vi "Create NIVS Custom Device API.vi"(8 "error in":errorcluster, 9 "Custom Device Item Ref":u64 format="%.0x") -> (0 "error out":errorcluster, 3 "NIVS Custom Device API out":refnum<class "NIVS Custom Device API.lvclass">)   [LabVIEW 2026, in "Template Engine.lvlib" / "NIVS Custom Device API.lvclass"]
uses:
  NIVS Custom Device API.lvclass
  NIVS Custom Device API.lvclass/NIVS Custom Device API.ctl
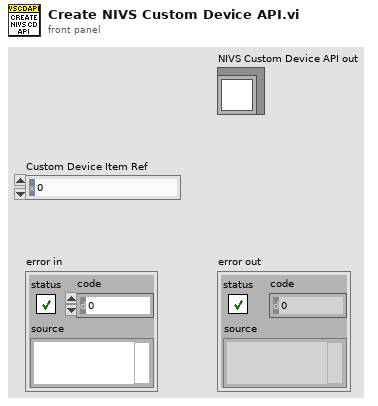
[diagram p1: front panel]
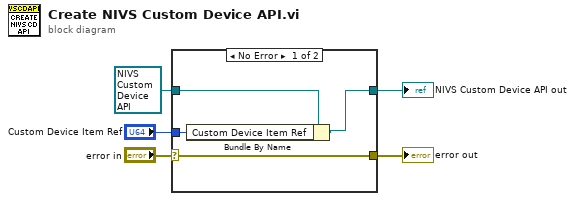
[diagram p0: block diagram]
diagram:
  n1 = case shown="No Error" "error in" {
    selector: "error in" -> [w9 w11]
    tunnel: [w9 w11] -> w4
    tunnel: [w6 w10] -> w1
    tunnel: refnum<class "NIVS Custom Device API.lvclass"> refnum ("VS Engine Plugin API in") -> [w7 w10]
    tunnel: "Custom Device Item Ref" -> [w8 _]
    frame No Error {
      n2 = Bundle By Name(cluster=w7, "Custom Device Item Ref"=w8) -> (w6:refnum<class "NIVS Custom Device API.lvclass">)
    }
    frame Error {
    }
  }
  "error out" <- w4
  "NIVS Custom Device API out" <- w1
